vi "SaveConfig.vi"(8 "error in (no error)":errorcluster, 11 "Microscope in":refnum<class "Microscope.lvclass">) -> (0 "error out":errorcluster, 3 "Microscope out":refnum<class "Microscope.lvclass">)   [LabVIEW 2020, in "Microscope.lvlib" / "Microscope.lvclass"]
uses:
  Microscope.lvclass
  Microscope.lvclass/Microscope.ctl
  Component/Device/Device/Device.lvclass
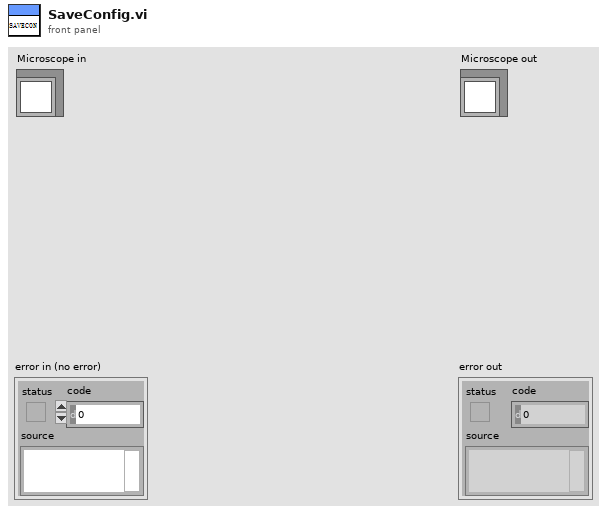
[diagram p1: front panel]
types:
  T1 = typedef "NI_LVConfig.lvlib/Config Data RefNum.ctl" = refnum<k1>
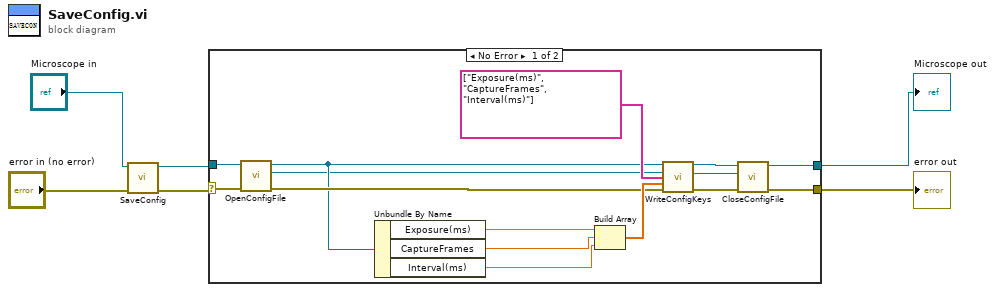
[diagram p0: block diagram]
diagram:
  n1 = call-parent "SaveConfig.vi"("error in (no error)"="error in (no error)", "GRMActor in"="Microscope in") -> ("error out"=w4:errorcluster, "GRMActor out"=w3:refnum<class "Microscope.lvclass">)  [unwired: 8 in]
  n2 = case shown="No Error" w4 {
    selector: w4 -> [w21 w22]
    tunnel: [w13 w22] -> w1
    tunnel: [w11 w23] -> w2
    tunnel: w3 -> [w10 w23]
    frame No Error {
      n3 = call-dynamic "OpenConfigFile.vi"("error in (no error)"=w21, "GRMActor in"=w10) -> ("error out"=w14:errorcluster, "refnum"=w8:T1, "GRMActor out"=w9:refnum<class "Microscope.lvclass">)  [unwired: 7 in]
      n4 = Unbundle By Name(w9) -> ("Exposure(ms)"=w18:dbl, "CaptureFrames"=w17:dbl, "Interval(ms)"=w16:dbl)
      n5 = Build Array(w18, w17, w16) -> (w15:dbl[])
      n6 = call-dynamic "WriteConfigKeys.vi"("GRMActor in"=w9, "Config Refnum"=w8, "Keys"=string[] ["Exposure(ms)", "CaptureFrames", "Interval(ms)"], "Value"=w15, "error in (no error)"=w14) -> ("GRMActor out"=w12:refnum<class "Microscope.lvclass">, "Config Refnum dup"=w7:T1, "error out"=w20:errorcluster)  [unwired: 8 in]
      n7 = call-dynamic "CloseConfigFile.vi"("error in (no error)"=w20, "refnum"=w7, "GRMActor in"=w12) -> ("error out"=w13:errorcluster, "GRMActor out"=w11:refnum<class "Microscope.lvclass">)  [unwired: 7 in]
    }
    frame Error {
    }
  }
  "error out" <- w1
  "Microscope out" <- w2
